vi "IO Write.vi"(10 "data":bool, 11 "I/O":refnum<k21>) -> ()   [LabVIEW 2017, in "HD44780 FPGA.lvlib"]
uses:
  HD44780 FPGA.lvlib
  <vilib>/rvi/eio/common/nirviEmuTemplateMethod_errors.vi
  <vilib>/eio/EIONode/EIONode.xnode
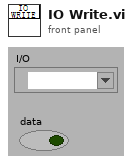
[diagram p1: front panel]
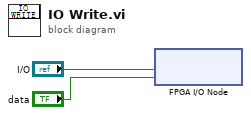
[diagram p0: block diagram]
diagram:
  n1 = xnode "FPGA I/O Node"("I/O Item"="data", "FPGA I/O In"="I/O") -> ()  [unwired: 1 out]
